vi "Test MQTT-4.7.1-2.vi"(8 "error in (no error)":errorcluster) -> (0 "error out":errorcluster)   [LabVIEW 2013]
uses:
  <vilib>/addons/_JKI Toolkits/Caraya/classes/Test/Test.lvclass
  <vilib>/addons/_JKI Toolkits/Caraya/classes/Assert/Assert.lvclass
  <vilib>/LabVIEW Open Source Project/MQTT Connection/MQTT_Base/TopicFilter/TopicFilter.lvclass
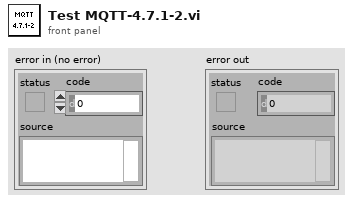
[diagram p1: front panel]
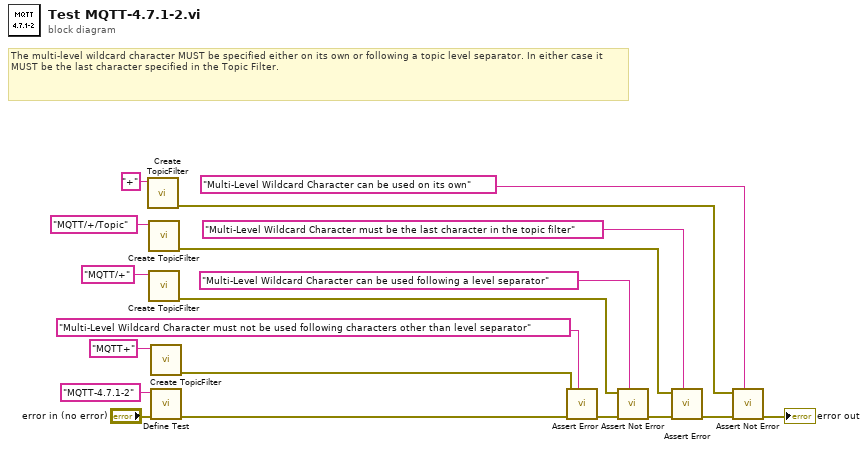
[diagram p0: block diagram]
diagram:
  # "The multi-level wildcard character MUST be specified either on its own or following a topic level separator. In either case it MUST be the last character specified in the Topic Filter."
  n1 = call <vilib>:"Create TopicFilter.vi"("Topic Filter"="+" ("Topic Name")) -> ("error out"=w7:errorcluster)  [unwired: 9 in, 1 out]
  n2 = call <vilib>:"Create TopicFilter.vi"("Topic Filter"="MQTT/+/Topic" ("Topic Name")) -> ("error out"=w2:errorcluster)  [unwired: 9 in, 1 out]
  n3 = call <vilib>:"Create TopicFilter.vi"("Topic Filter"="MQTT/+" ("Topic Name")) -> ("error out"=w3:errorcluster)  [unwired: 9 in, 1 out]
  n4 = call <vilib>:"Create TopicFilter.vi"("Topic Filter"="MQTT+" ("Topic Name")) -> ("error out"=w1:errorcluster)  [unwired: 9 in, 1 out]
  n5 = call <vilib>:"Define Test.vi"("error in (no error)"="error in (no error)", "Label (VI Title)"="MQTT-4.7.1-2") -> ("error out"=w16:errorcluster)  [unwired: 9 in]
  n6 = call <vilib>:"Assert Error.vi"("Label"="Multi-Level Wildcard Character must not be used following characters other than level separator", "error in (no error)"=w16, "Error?"=w1) -> ("error out"=w12:errorcluster)  [unwired: 8 in]
  n7 = call <vilib>:"Assert Not Error.vi"("Label"="Multi-Level Wildcard Character can be used following a level separator", "error in (no error)"=w12, "Not Error?"=w3) -> ("error out"=w11:errorcluster)  [unwired: 8 in]
  n8 = call <vilib>:"Assert Error.vi"("Label"="Multi-Level Wildcard Character must be the last character in the topic filter", "error in (no error)"=w11, "Error?"=w2) -> ("error out"=w14:errorcluster)  [unwired: 8 in]
  n9 = call <vilib>:"Assert Not Error.vi"("Label"="Multi-Level Wildcard Character can be used on its own", "error in (no error)"=w14, "Not Error?"=w7) -> ("error out"=→"error out":errorcluster)  [unwired: 8 in]
